vi "Windows_App.vi"() -> ()   [LabVIEW 2015]
uses:
  C:/Program Files (x86)/National Instruments/LabVIEW 2015/examples/Instrument IO/Serial/support/Serial - Settings.ctl
  <vilib>/Instr/_visa.llb/VISA Configure Serial Port (Instr).vi
panel:
  out "Values":dbl[](array[numeric])=[1.0, 1.0, 1.0, 1.0, 1.0, 1.0, 1.0, 1.0, 1.0, 1.0, 1.0, 1.0, 1.0] format="%_6g"
  out "String":string="4000\t4000\t4000\t4000\t4000\t4000\t4000\t4000\t4000\t4000\t4000\t4000\t4000\r\n"
  in  "Attenuations":dbl[](array[slide])=[1.0, 1.0, 1.0, 1.0, 1.0, 1.0, 1.0, 1.0, 1.0, 1.0, 1.0, 1.0, 1.0] scale=0.0..1.0
  in  "VISA resource name":refnum<visa-resource-name>="COM9"
  in  "Serial Settings":T1={"baud rate"=9600, "data bits"=8, "parity"=enum."None", "stop bits"=10, "flow control"=0} {"flow control" items=["None"=0, "XON/XOFF"=1, "RTS/CTS"=2, "DTR/DSR"=4]; "stop bits" items=["1.0"=10, "1.5"=15, "2.0"=20]; "data bits" min=5 max=8 step=1; "baud rate" items=["75"=75, "110"=110, "134"=134, "150"=150, "300"=300, "600"=600, "1200"=1200, "1800"=1800, "2400"=2400, "4800"=4800, "7200"=7200, "9600"=9600, "14400"=14400, "19200"=19200, "28800"=28800, "38400"=38400, "56000"=56000, "57600"=57600, "115200"=115200, "128000"=128000, "230400"=230400]}
  in  "Stop":bool
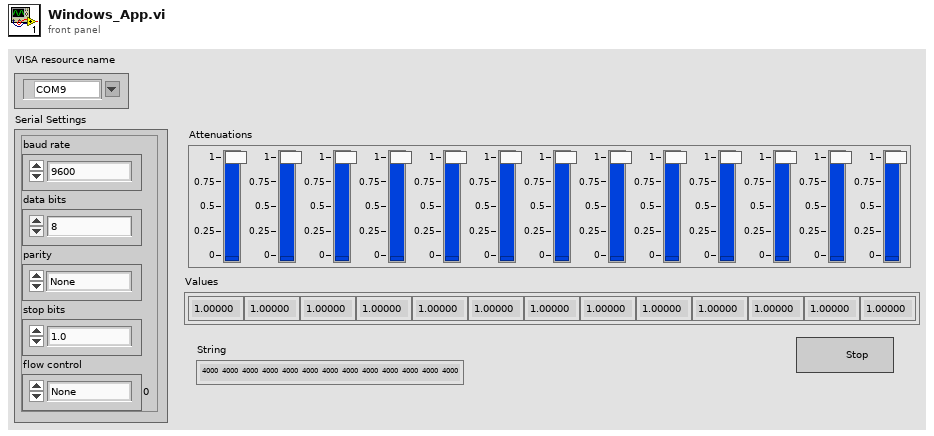
[diagram p1: front panel]
types:
  T1 = typedef "Serial - Settings.ctl" = cluster{"baud rate":u32, "data bits":u16, "parity":enum16{"None", "Odd", "Even", "Mark", "Space"}, "stop bits":u16, "flow control":u16}
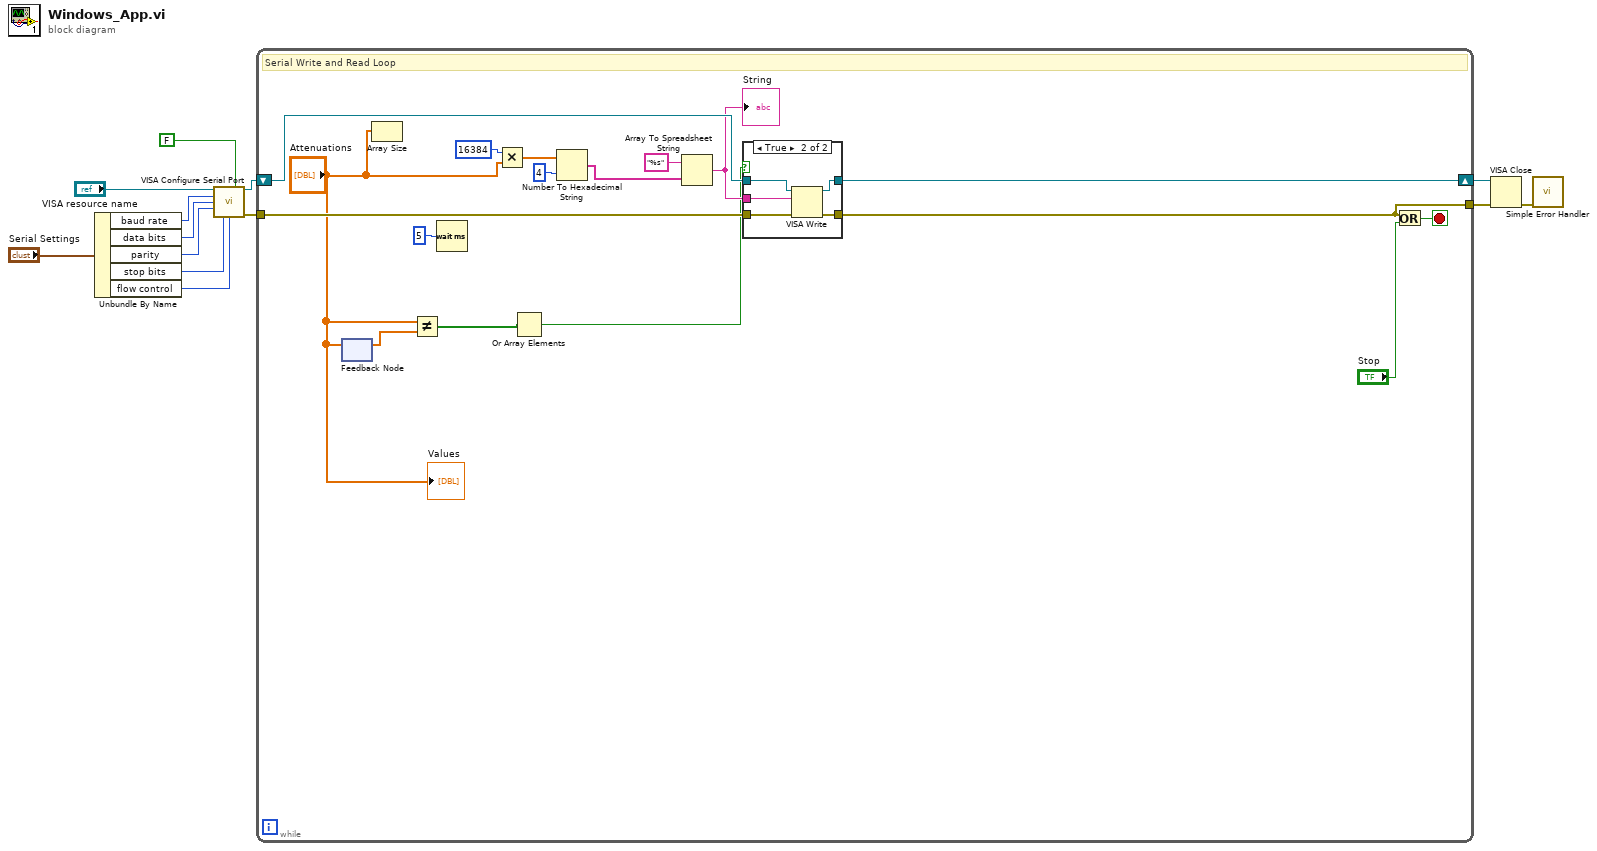
[diagram p0: block diagram]
diagram:
  n1 = Unbundle By Name("Serial Settings") -> ("baud rate"=w9:u32, "data bits"=w10:u16, "parity"=w11:enum16{"None", "Odd", "Even", "Mark", "Space"}, "stop bits"=w12:u16, "flow control"=w4:u16)
  n2 = call-poly "VISA Configure Serial Port"("VISA resource name"="VISA resource name", "Enable Termination\nChar (T)"=FALSE, "baud rate (9600)"=w9, "data bits (8)"=w10, "parity (0:none)"=w11, "stop bits (10: 1 bit)"=w12, "flow control (0:none)"=w4) -> ("VISA resource name out"=w3:refnum<visa-resource-name>, "error out"=w2:errorcluster)  [unwired: 3 in, 4 out]
  n3 = while {
    shift-right: [w19] -> w5
    shift-left: w3 -> [w30]
    tunnel: w2 -> [w29]
    tunnel: [w18] -> w6
    stop <- w27 stop-if-true
    # "Serial Write and Read Loop"
    n4 = feedback #1() -> (w17:dbl[])  [unwired: 1 in]
    n5 = feedback-in #1("Attenuations") -> ()
    n6 = Array Size(array="Attenuations") -> ()  [unwired: 1 out]
    n7 = Not Equal?(x="Attenuations", y=w17) -> (x != y?=w16:bool[])
    n8 = Wait (ms)(milliseconds to wait=u32 5) -> ()  [unwired: 1 out]
    n9 = Multiply(x=16384, y="Attenuations") -> (x*y=w22:dbl[])
    n10 = Or Array Elements(Boolean array=w16) -> (logical OR=w15:bool)
    n11 = Number To Hexadecimal String(1:4, 2:w22) -> (0:w20:string[])
    n12 = Array To Spreadsheet String(array=w20, 3:"%s") -> (spreadsheet string=w24:string)  [unwired: 1 in]
    "String" <- w24
    n13 = case shown="True" w15 {
      tunnel: w30 -> [w32 w37]
      tunnel: w29 -> [w31 w36]
      tunnel: [w32 w35] -> w19
      tunnel: [w31 w34] -> w18
      tunnel: w24 -> [_ w33]
      frame False {
      }
      frame True {
        n14 = VISA Write(VISA resource name=w37, write buffer=w33, error in (no error)=w36) -> (VISA resource name out=w35:refnum<visa-resource-name>, error out=w34:errorcluster)  [unwired: 1 out]
      }
    }
    n15 = Or(x=w18, y="Stop") -> (x .or. y?=w27:bool)
    "Values" <- "Attenuations"
  }
  n16 = VISA Close(VISA resource name=w5, error in (no error)=w6) -> (error out=w7:errorcluster)
  n17 = call <vilib>:"Simple Error Handler.vi"("error in (no error)"=w7) -> ()  [unwired: 1 in, 8 out]
